vi "ui_DataLog Get or Query Subset.vi"(0 "database":string, 7 "subset name in (query)":string, 11 "error in (no error)":errorcluster) -> (4 "OK?":bool, 8 "subset name out":string, 10 "tags in subset":string[](array[string]), 15 "error out":errorcluster)   [LabVIEW 2012]
doc: "Gets a specified tag subset or, if no such subset is found, queries it via a dialog that lists the subset names."
uses:
  served/DataLog Database Infos_srv.ctl
  typedefs/t_DataLog Tag Info List Methods.ctl
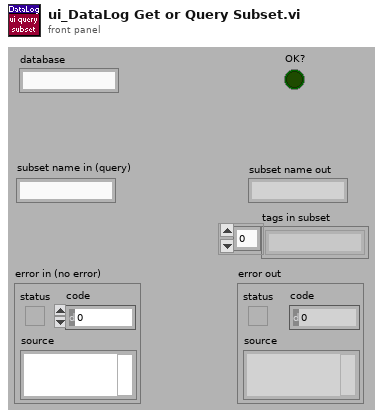
[diagram p1: front panel]
types:
  T1 = typedef "t_DataLog Tag Info List Methods.ctl" = enum16{"initialize", "create", "create empty", "rename", "delete", "test tag", "get", "get by name", "get default", "get list", "get path", "get subsets", "set subsets", "set config", "set capacity", "#tags", "go live", "set unlocked", "set mirrored"}
  T2 = typedef "DataLog Database Infos_srv.ctl" = refnum<vi>
  T3 = typedef "t_DataLog Tag Subset.ctl" = cluster{"name":string, "tags":string[]}
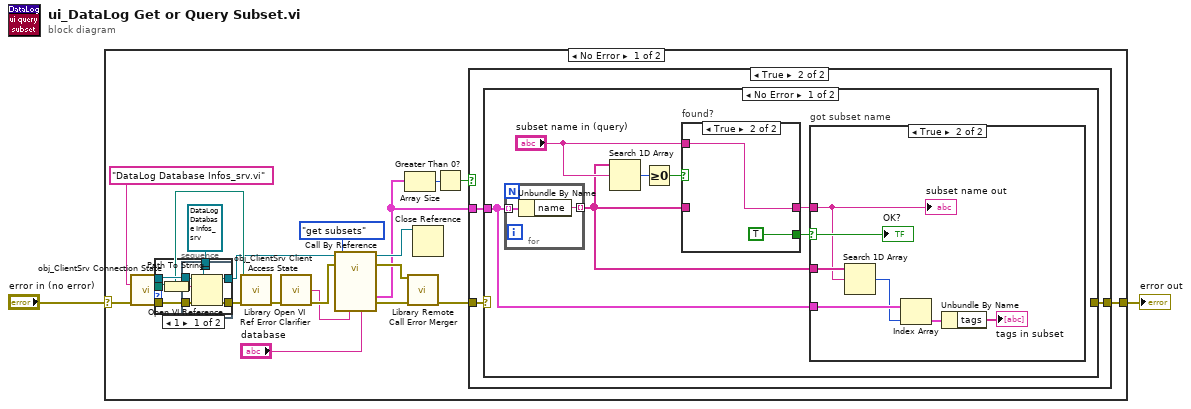
[diagram p0: block diagram]
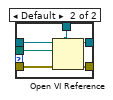
[diagram p2: hidden frame]
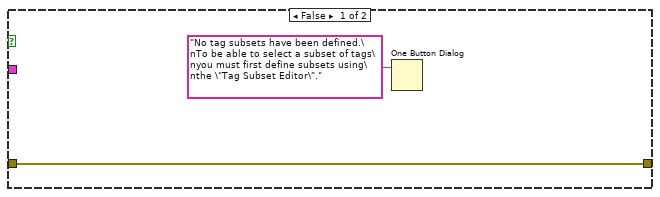
[diagram p3: hidden frame]
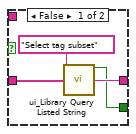
[diagram p5: hidden frame]
diagram:
  n1 = case shown="No Error" "error in (no error)" {
    selector: "error in (no error)" -> [w15 w73]
    tunnel: [w16 w73] -> w2
    frame No Error {
      n2 = call "obj_ClientSrv Connection State.vi"("machine{connect}/VI{get state} name (local/no path resolution)"="DataLog Database Infos_srv.vi", "error in (no error)"=w15) -> ("server app ref"=w6:refnum<vi>, "resolved server path"=w5:path, "error out"=w7:errorcluster)  [unwired: 6 in, 5 out]
      n3 = stacked-sequence {
        tunnel: [w29] -> w4
        tunnel: [w28] -> w8
        tunnel: w7 -> [w27]
        tunnel: w6 -> [w26]
        tunnel: w5 -> [w25]
        tunnel: T2 refnum ("database infos") -> [w24]
        frame #0 {
          # "avoid LV8 complaints"
          n4 = Path to Array of Strings(0:w25) -> (2:w30:string[])  [unwired: 1 out]
          n5 = Array Size(array=w30) -> (size(s)=w31:i32)
          n6 = case shown="1" w31 {
            tunnel: w25 -> [w38 w44]
            tunnel: w26 -> [w36 w43]
            tunnel: [w34 w39] -> w29
            tunnel: [w32 w42] -> w28
            tunnel: w24 -> [w33 w41]
            tunnel: w27 -> [w35 w40]
            frame 1 {
              n7 = Path To String(path=w38) -> (string=w37:string)
              n8 = Open VI Reference(type specifier VI Refnum (for type only)=w33, application reference (local)=w36, vi path=w37, error in (no error)=w35) -> (vi reference=w34:T2, error out=w32:errorcluster)  [unwired: 2 in]
            }
            frame Default {
              n9 = Open VI Reference(type specifier VI Refnum (for type only)=w41, application reference (local)=w43, vi path=w44, error in (no error)=w40) -> (vi reference=w39:T2, error out=w42:errorcluster)  [unwired: 2 in]
            }
          }
        }
      }
      n10 = call "Library Open VI Ref Error Clarifier.vi"("VI path"=w5, "called VI error (no error)"=w8) -> ("error out"=w18:errorcluster)  [unwired: 13 in]
      n11 = call "obj_ClientSrv Client Access State.vi"("error in (no error)"=w18) -> ("certificate"=w11:string, "error out"=w23:errorcluster)  [unwired: 13 in]
      n12 = call-by-ref "?"(reference=w4, error in=w23, "method"=t_DataLog_Tag_Info_List_Methods."get subsets", "certificate in"=w11, "database (current)"="database") -> (reference out=w22:T2, error out=w21:errorcluster, "subsets out"=w12:T3[], 15:"error out"=w20:errorcluster)  [unwired: 7 in, 4 out]
      n13 = Array Size(array=w12) -> (size(s)=w14:i32)
      n14 = call "Library Remote Call Error Merger.vi"("call by reference node error"=w21, "called VI error (no error)"=w20) -> ("error out"=w17:errorcluster)  [unwired: 13 in]
      n15 = Close Reference(reference=w22) -> ()  [unwired: 1 in, 1 out]
      n16 = Greater Than 0?(x=w14) -> (x > 0?=w13:bool)
      n17 = case shown="True" w13 {
        tunnel: w12 -> [_ w49]
        tunnel: w17 -> [w46 w48]
        tunnel: [w46 w47] -> w16
        frame False {
          n18 = One Button Dialog(message="No tag subsets have been defined.\nTo be able to select a subset of tags\nyou must first define subsets using\nthe \"Tag Subset Editor\".") -> ()  [unwired: 1 in, 1 out]
        }
        frame True {
          n19 = case shown="No Error" w48 {
            selector: w48 -> [_ w72]
            tunnel: w49 -> [w56 _]
            tunnel: [_ w72] -> w47
            frame No Error {
              n20 = for {
                tunnel: [w71] -> w50 mode=indexing
                tunnel: w56 -> [w70] mode=indexing
                n21 = Unbundle By Name(w70) -> ("name"=w71:string)
              }
              n22 = Search 1D Array(1D array=w50, element="subset name in (query)") -> (index of element=w53:i32)  [unwired: 1 in]
              n23 = Greater Or Equal To 0?(x=w53) -> (x >= 0?=w52:bool)
              n24 = case "found?" shown="True" w52 {
                tunnel: w50 -> [w67 _]
                tunnel: [w66 w68] -> w54
                tunnel: [w64 TRUE ("OKed?")] -> w55
                tunnel: "subset name in (query)" -> [_ w68]
                frame False {
                  n25 = call "ui_Library Query Listed String.vi"("prompt"="Select tag subset", "list of strings"=w67) -> ("OKed?"=w64:bool, "selected string"=w66:string)  [unwired: 12 in]
                }
                frame True {
                }
              }
              n26 = case "got subset name" shown="True" w55 {
                selector: w55 -> [_ w60]
                tunnel: w56 -> [_ w63]
                tunnel: w54 -> [_ w58]
                tunnel: w50 -> [_ w59]
                frame False {
                }
                frame True {
                  n27 = Search 1D Array(1D array=w59, element=w58) -> (index of element=w57:i32)  [unwired: 1 in]
                  n28 = Index Array(array=w63, index=w57) -> (element=w62:T3)
                  n29 = Unbundle By Name(w62) -> ("tags"=→"tags in subset":string[])
                  "OK?" <- w60
                  "subset name out" <- w58
                }
              }
            }
            frame Error {
            }
          }
        }
      }
    }
    frame Error {
    }
  }
  "error out" <- w2
